vi "All channel sine fitting.vi"(4 "error in":errorcluster, 5 "dt":dbl=1.0, 6 "LM fitting?":bool=TRUE, 7 "scaled data array":T1[](array[typedef])) -> (0 "error out":errorcluster, 1 "Fit":cluster{dbl[], "best nonlinear fit":dbl[]}[](graph), 2 "Raw":cluster{dbl[], dbl[]}[](graph), 3 "best fit parameters":dbl[][](array[numeric]))   [LabVIEW 2020, in "Measure angular gains.lvlib"]
uses:
  Measure angular gains.lvlib
  SignalConversion/ScaledData.ctl
  SignalConversion/Measrured TrapXYZ.ctl
  SignalConversion/Data Before Angle Compensation.ctl
  SignalConversion/Angle compensated data.ctl
  SignalConversion/XYZ Signals.ctl
  SignalConversion/Set TrapXYZ.ctl
  SignalConversion/SignalConverson.lvlib
panel:
  out "Now Is Fitting Curve: 2":i32
  out "Fit 2":cluster{dbl[], "best nonlinear fit":dbl[]}[](graph)
  out "Now Is Fitting Curve:":i32
  # "y0\nfreq\namp\nphase\nresidue"
  # "Channel Info:\nA, D, Power P, Power S, L, R, Vsum, Vx, Vy"
  # "a0+a2*sin(x*6.2832*a1+a3)"
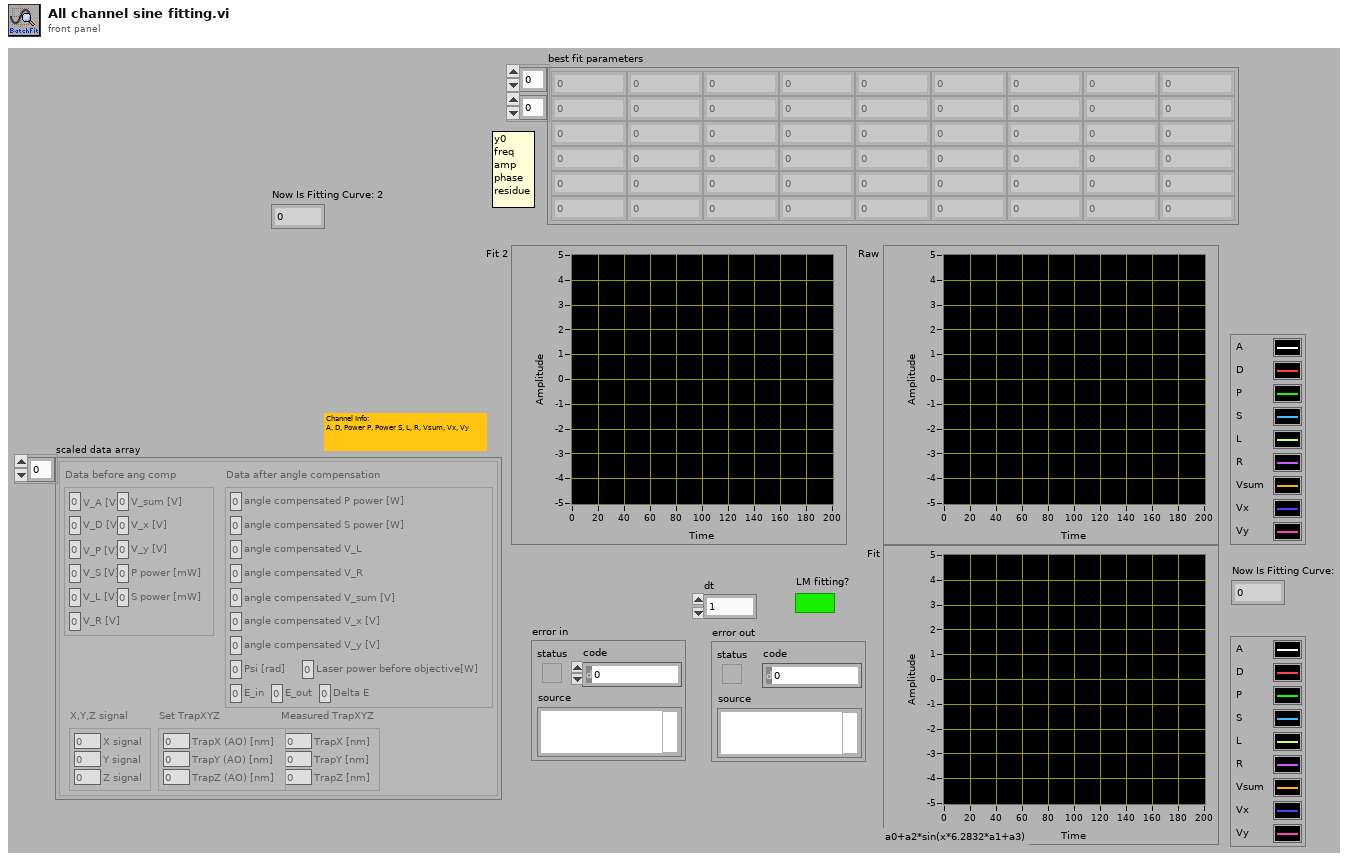
[diagram p1: front panel]
types:
  T1 = typedef "SignalConverson.lvlib/ScaledData.ctl" = cluster{"Measured TrapXYZ":T2, "Data before ang comp":T3, "Data after angle compensation":T4, "X,Y,Z signal":T5, "Set TrapXYZ":T6}
  T2 = typedef "SignalConverson.lvlib/Measrured TrapXYZ.ctl" = cluster{"TrapX [nm]":dbl, "TrapY [nm]":dbl, "TrapZ [nm]":dbl}
  T3 = typedef "SignalConverson.lvlib/Data Before Angle Compensation.ctl" = cluster{"V_A [V]":dbl, "V_D [V]":dbl, "V_P [V]":dbl, "V_S [V]":dbl, "V_L [V]":dbl, "V_R [V]":dbl, "V_sum [V]":dbl, "V_x [V]":dbl, "V_y [V]":dbl, "P power [mW]":dbl, "S power [mW]":dbl}
  T4 = typedef "SignalConverson.lvlib/Angle compensated data.ctl" = cluster{"angle compensated P power [W]":dbl, "angle compensated S power [W]":dbl, "angle compensated V_L":dbl, "angle compensated V_R":dbl, "angle compensated V_sum [V]":dbl, "angle compensated V_x [V]":dbl, "angle compensated V_y [V]":dbl, "Psi [rad]":dbl, "Laser power before objective[W]":dbl, "E_in":dbl, "E_out":dbl, "Delta E":dbl}
  T5 = typedef "SignalConverson.lvlib/XYZ Signals.ctl" = cluster{"X signal":dbl, "Y signal":dbl, "Z signal":dbl}
  T6 = typedef "SignalConverson.lvlib/Set TrapXYZ.ctl" = cluster{"TrapX (AO) [nm]":dbl, "TrapY (AO) [nm]":dbl, "TrapZ (AO) [nm]":dbl}
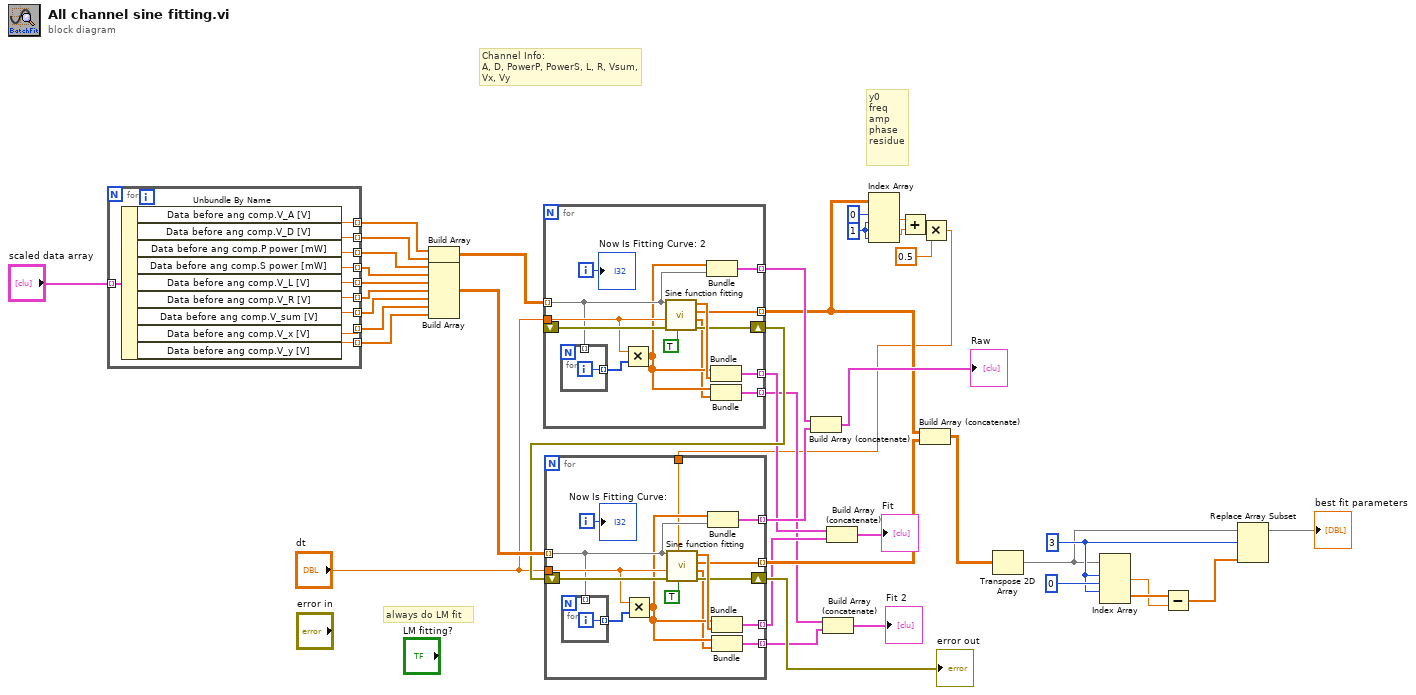
[diagram p0: block diagram]
diagram:
  w7 = 1 ("index (row)")
  w37 = 3 ("index (row)")
  # "y0\nfreq\namp\nphase\nresidue"
  # "always do LM fit"
  # "Channel Info:\nA, D, PowerP, PowerS, L, R, Vsum, Vx, Vy"
  n1 = for {
    tunnel: "scaled data array" -> [w42] mode=indexing
    tunnel: [w51] -> w25 mode=indexing
    tunnel: [w50] -> w24 mode=indexing
    tunnel: [w49] -> w33 mode=indexing
    tunnel: [w48] -> w32 mode=indexing
    tunnel: [w47] -> w31 mode=indexing
    tunnel: [w46] -> w30 mode=indexing
    tunnel: [w45] -> w29 mode=indexing
    tunnel: [w44] -> w28 mode=indexing
    tunnel: [w43] -> w27 mode=indexing
    n2 = Unbundle By Name(w42) -> ("Data before ang comp.V_A [V]"=w51:dbl, "Data before ang comp.V_D [V]"=w50:dbl, "Data before ang comp.P power [mW]"=w49:dbl, "Data before ang comp.S power [mW]"=w48:dbl, "Data before ang comp.V_L [V]"=w47:dbl, "Data before ang comp.V_R [V]"=w46:dbl, "Data before ang comp.V_sum [V]"=w45:dbl, "Data before ang comp.V_x [V]"=w44:dbl, "Data before ang comp.V_y [V]"=w43:dbl)
  }
  n3 = Build Array(w25, w24) -> (w21:dbl[][])
  n4 = Build Array(w33, w32, w31, w30, w29, w28, w27) -> (w26:dbl[][])
  n5 = for {
    tunnel: w21 -> [w57] mode=indexing
    tunnel: [w56] -> w9 mode=indexing
    tunnel: [w64] -> w15 mode=indexing
    shift-right: [w61] -> w23
    shift-left: _ -> [w62]
    tunnel: "dt" -> [w60]
    tunnel: [w58] -> w16 mode=indexing
    tunnel: [w53] -> w10 mode=indexing
    i -> [w65]
    n6 = for {
      tunnel: [w66] -> w59 mode=indexing
      tunnel: w57 -> [_] mode=indexing
      i -> [w66]
    }
    n7 = Multiply(x=w60, y=w59) -> (x*y=w55:dbl[])
    n8 = call "Sine function fitting.vi"("Additional\nLM fitting?"=TRUE ("Additional\nLM fitting?"), "error in (no error)"=w62, "dt"=w60, "Input Y"=w57) -> ("error out"=w61:errorcluster, "Residue"=w54:dbl[], "best fit parameters"=w56:dbl[], "best nonlinear fit"=w63:dbl[])  [unwired: 4 in]
    n9 = Bundle(w55, w57) -> (w58:cluster{dbl[], dbl[]})  [unwired: 1 in]
    n10 = Bundle(w55, "best nonlinear fit"=w63) -> (w64:cluster{dbl[], "best nonlinear fit":dbl[]})  [unwired: 1 in]
    n11 = Bundle(w55, "Residue"=w54) -> (w53:cluster{dbl[], "Residue":dbl[]})  [unwired: 1 in]
    "Now Is Fitting Curve: 2" <- w65
  }
  n12 = Index Array(array=w9, index (row) #1=0 ("index (row)"), index (col) #1=w7, index (row) #2=w7, index (col) #2=w7) -> (element #1=w5:dbl, element #2=w6:dbl)
  n13 = Add(x=w5, y=w6) -> (x+y=w4:dbl)
  n14 = Multiply(x=w4, y=0.5) -> (x*y=w2:dbl)
  n15 = for {
    tunnel: w26 -> [w73] mode=indexing
    tunnel: [w72] -> w20 mode=indexing
    tunnel: [w80] -> w14 mode=indexing
    shift-right: [w77] -> w41
    shift-left: w23 -> [w78]
    tunnel: "dt" -> [w76]
    tunnel: [w74] -> w17 mode=indexing
    tunnel: [w69] -> w11 mode=indexing
    tunnel: w2 -> [w67]
    i -> [w81]
    n16 = for {
      tunnel: [w82] -> w75 mode=indexing
      tunnel: w73 -> [_] mode=indexing
      i -> [w82]
    }
    n17 = Multiply(x=w76, y=w75) -> (x*y=w71:dbl[])
    n18 = call "Sine function fitting.vi"("Additional\nLM fitting?"=TRUE ("Additional\nLM fitting?"), "frequency guess"=w67, "error in (no error)"=w78, "dt"=w76, "Input Y"=w73) -> ("error out"=w77:errorcluster, "Residue"=w70:dbl[], "best fit parameters"=w72:dbl[], "best nonlinear fit"=w79:dbl[])  [unwired: 3 in]
    n19 = Bundle(w71, w73) -> (w74:cluster{dbl[], dbl[]})  [unwired: 1 in]
    n20 = Bundle(w71, "best nonlinear fit"=w79) -> (w80:cluster{dbl[], "best nonlinear fit":dbl[]})  [unwired: 1 in]
    n21 = Bundle(w71, "Residue"=w70) -> (w69:cluster{dbl[], "Residue":dbl[]})  [unwired: 1 in]
    "Now Is Fitting Curve:" <- w81
  }
  "error out" <- w41
  n22 = Build Array (concatenate)(w16, w17) -> (→"Raw":cluster{dbl[], dbl[]}[])
  n23 = Build Array (concatenate)(w10, w11) -> (→"Fit 2":cluster{dbl[], "Residue":dbl[]}[])
  n24 = Build Array (concatenate)(w15, w14) -> (→"Fit":cluster{dbl[], "best nonlinear fit":dbl[]}[])
  n25 = Build Array (concatenate)(w9, w20) -> (w19:dbl[][])
  n26 = Transpose 2D Array(2D array=w19) -> (transposed array=w35:dbl[][])
  n27 = Index Array(array=w35, index (row) #1=w37, index (col) #1=0 ("disabled index (col)"), index (row) #2=w37) -> (element #1=w38:dbl, element #2=w39:dbl[])  [unwired: 1 in]
  n28 = Subtract(x=w39, y=w38) -> (x-y=w36:dbl[])
  n29 = Replace Array Subset(array=w35, new element=w36, index (row)=w37) -> (→"best fit parameters":dbl[][])  [unwired: 1 in]
